vi "Waveform_from_duty_cycle.vi"(9 "Duty cycle":dbl, 10 "Step samples":i32, 11 "Total samples":i32) -> (3 "odour waveform array":bool[](array[boolean]))   [LabVIEW 2016]
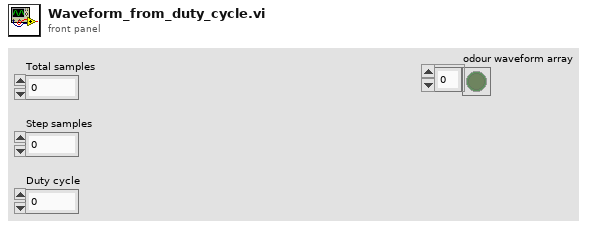
[diagram p1: front panel]
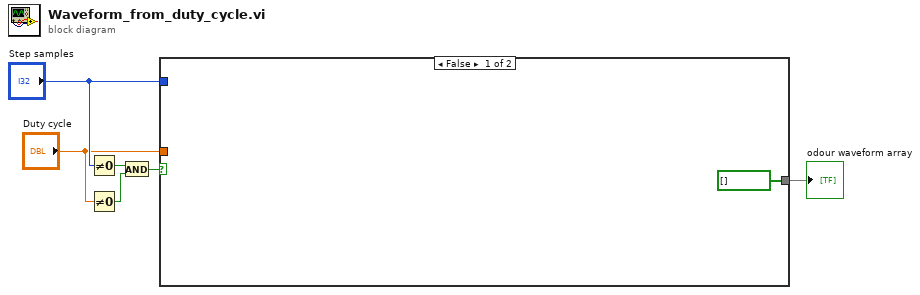
[diagram p0: block diagram]
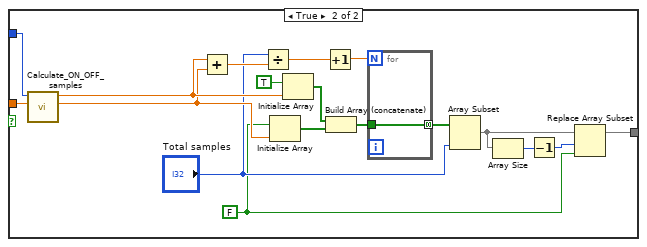
[diagram p2: hidden frame]
diagram:
  n1 = Not Equal To 0?(x="Step samples") -> (x != 0?=w3:bool)
  n2 = Not Equal To 0?(x="Duty cycle") -> (x != 0?=w2:bool)
  n3 = And(x=w3, y=w2) -> (x .and. y?=w1:bool)
  n4 = case shown="False" w1 {
    tunnel: "Step samples" -> [_ w25]
    tunnel: "Duty cycle" -> [_ w24]
    tunnel: [bool[] [] w8] -> w6
    frame False {
    }
    frame True {
      w9 = FALSE
      n5 = call "Calculate_ON_OFF_samples.vi"("Duty cycle"=w24, "Step samples"=w25) -> ("OFF samples"=w18:dbl, "ON samples"=w19:dbl)  [unwired: 8 in]
      n6 = Add(x=w19, y=w18) -> (x+y=w17:dbl)
      n7 = Divide(x="Total samples", y=w17) -> (x/y=w16:dbl)
      n8 = Initialize Array(w9, w18) -> (w22:bool[])
      n9 = Initialize Array(TRUE, w19) -> (w21:bool[])
      n10 = Increment(x=w16) -> (x+1=w15:dbl)
      n11 = Build Array (concatenate)(w21, w22) -> (w20:bool[])
      n12 = for {
        N: w15 -> [_]
        tunnel: w20 -> [w26]
        tunnel: [w26] -> w14 mode=concatenating
      }
      n13 = Array Subset(array=w14, length="Total samples") -> (w12:bool[])  [unwired: 1 in]
      n14 = Array Size(array=w12) -> (size(s)=w11:i32)
      n15 = Decrement(x=w11) -> (x-1=w10:i32)
      n16 = Replace Array Subset(array=w12, new element=w9, index=w10) -> (w8:bool[])
    }
  }
  "odour waveform array" <- w6
